vi "DMA Timeout (SubVI).vi"(11 "Timeout":bool) -> (3 "DMA Timeout":bool)   [LabVIEW 2015]
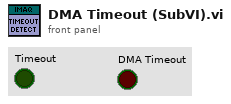
[diagram p1: front panel]
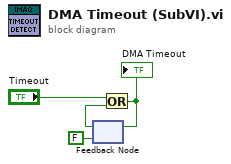
[diagram p0: block diagram]
diagram:
  n1 = feedback #1(FALSE) -> (w2:bool)
  n2 = Or(x="Timeout", y=w2) -> (x .or. y?=w3:bool)
  "DMA Timeout" <- w3
  n3 = feedback-in #1(w3) -> ()
